vi "CheckRemoteControl.vi"(0 "Universal Robot.lvclass in":refnum<class "Universal Robot.lvclass">, 5 "error in (no error)":errorcluster) -> (14 "Universal Robot.lvclass out":refnum<class "Universal Robot.lvclass">, 19 "error out":errorcluster)   [LabVIEW 2016, in "Universal Robot.lvclass"]
uses:
  Universal Robot.lvclass
  Universal Robot.lvclass/Universal Robot.ctl
  Client Interfaces/Dashboard Server/Dashboard Server.lvclass
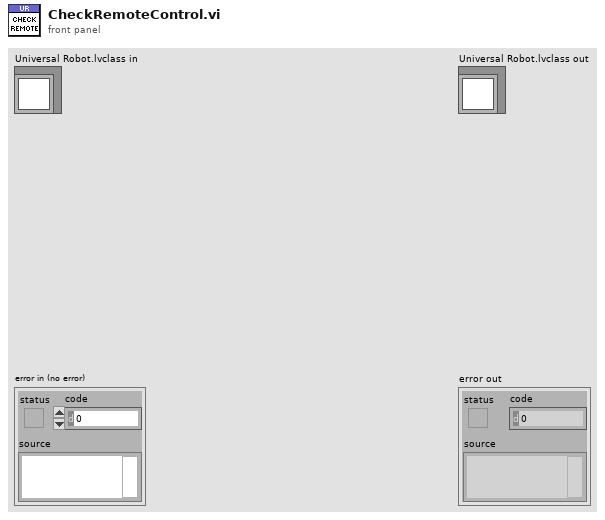
[diagram p1: front panel]
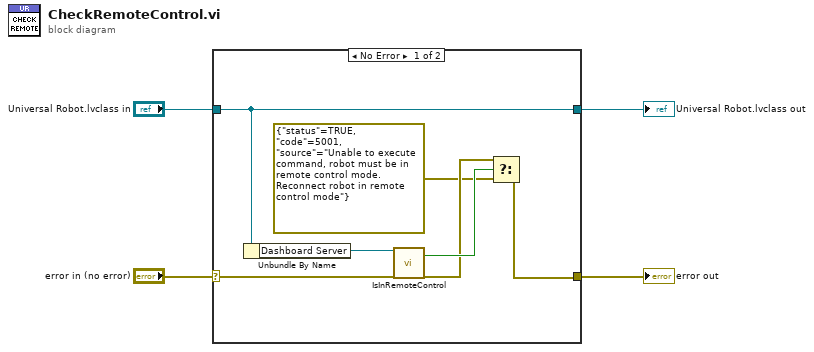
[diagram p0: block diagram]
diagram:
  n1 = case shown="No Error" "error in (no error)" {
    selector: "error in (no error)" -> [w9 w13]
    tunnel: [w6 w13] -> w3
    tunnel: "Universal Robot.lvclass in" -> [w11 w12]
    tunnel: [w11 w12] -> w1
    frame No Error {
      n2 = Unbundle By Name(w11) -> ("Dashboard Server"=w10:refnum<class "Dashboard Server.lvclass">)
      n3 = call-dynamic "IsInRemoteControl.vi"("DashboardServer in"=w10, "error in (no error)"=w9) -> ("remoteControl"=w8:bool, "error out"=w7:errorcluster)  [unwired: 15 in, 1 out]
      n4 = Select(t=w7, s=w8, f=errorcluster {"status"=TRUE, "code"=5001, "source"="Unable to execute command, robot must be in remote control mode. Reconnect robot in remote control mode"} ("error constant")) -> (s? t:f=w6:errorcluster)
    }
    frame Error {
    }
  }
  "error out" <- w3
  "Universal Robot.lvclass out" <- w1
